vi "UMLEditor BusyDialog.vi"(1 "ToDialog":refnum<user-event>, 2 "FromDialog":refnum<queue>, 5 "error in":errorcluster) -> (19 "error out":errorcluster)   [LabVIEW 2012]
panel:
  out "StatusOut":string
  in  "Abort":bool
  out "TitleOut":string
  out "LoadedVIs":i32(graph)
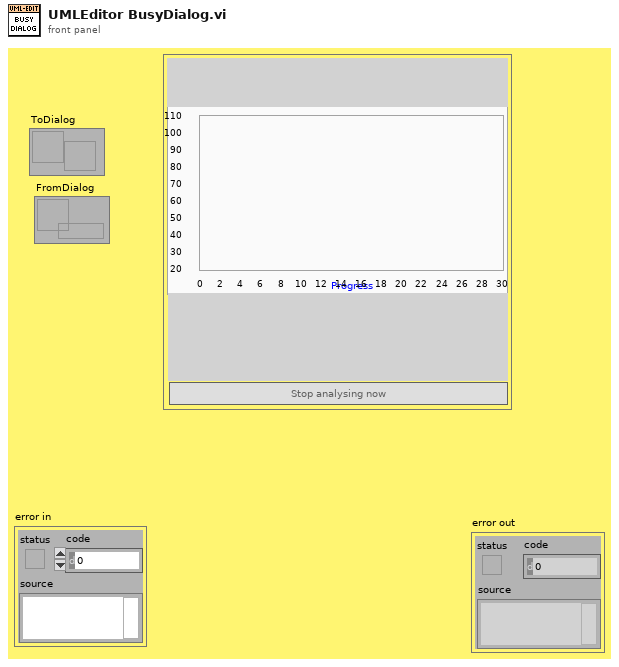
[diagram p1: front panel]
types:
  T1 = cluster{"CommandArgument":string, "Active":bool, "VIsInMem":i32, "ShowVIs":bool, "Event":refnum<event-registration>}
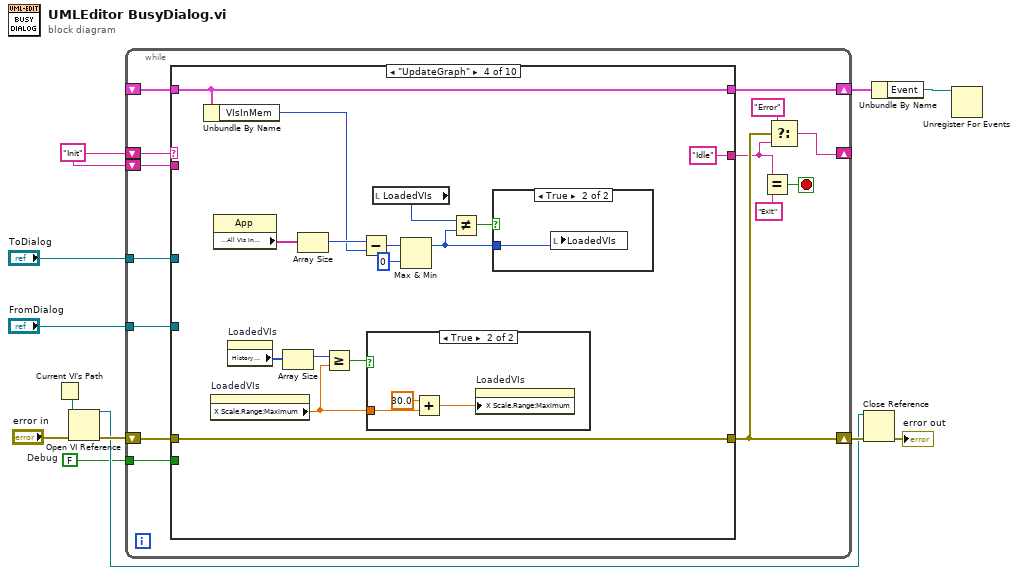
[diagram p0: block diagram]
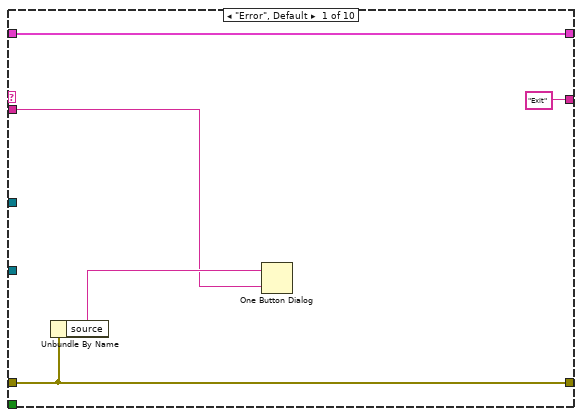
[diagram p2: hidden frame]
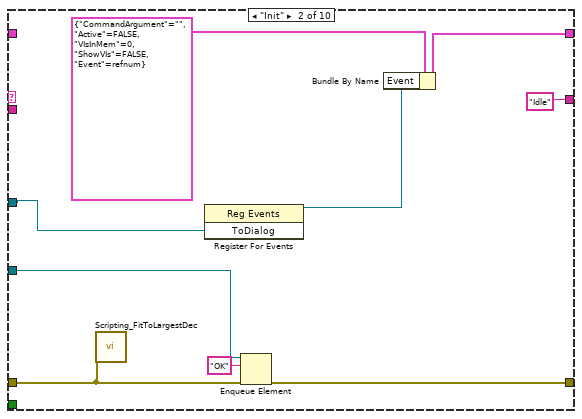
[diagram p3: hidden frame]
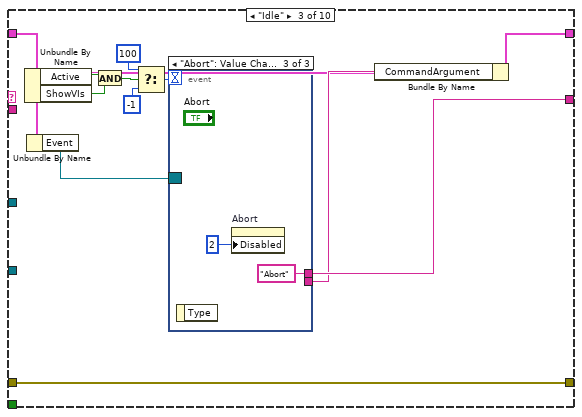
[diagram p4: hidden frame]
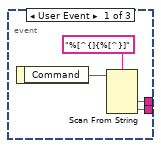
[diagram p5: hidden frame]
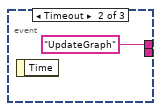
[diagram p6: hidden frame]
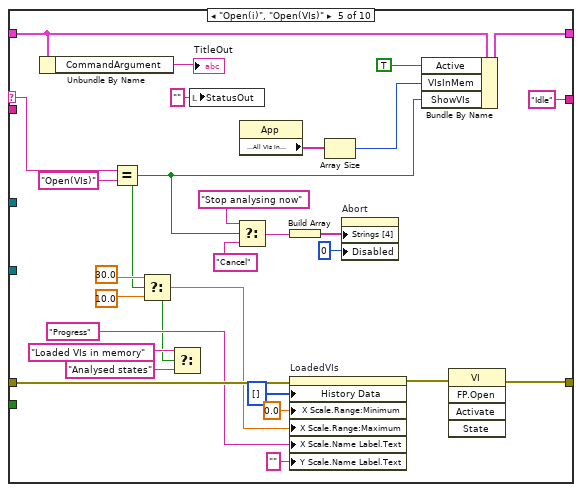
[diagram p9: hidden frame]
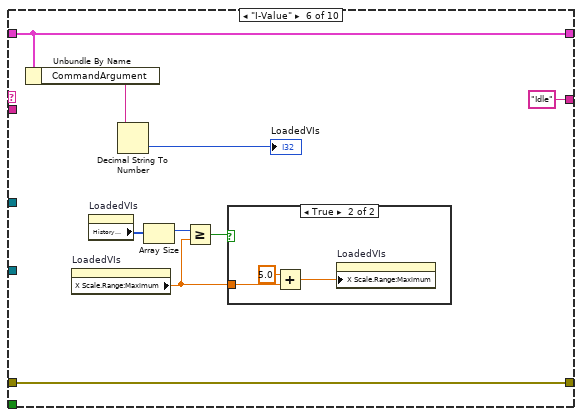
[diagram p10: hidden frame]
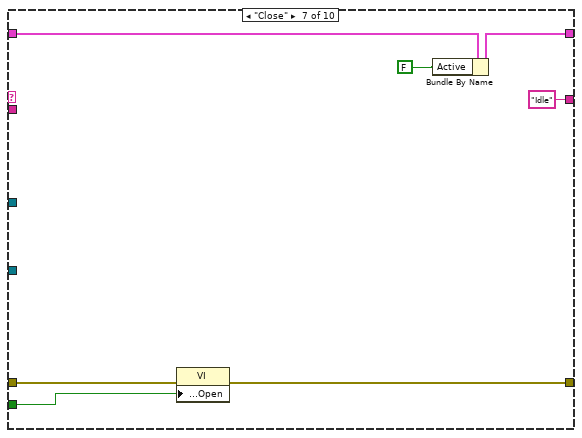
[diagram p12: hidden frame]
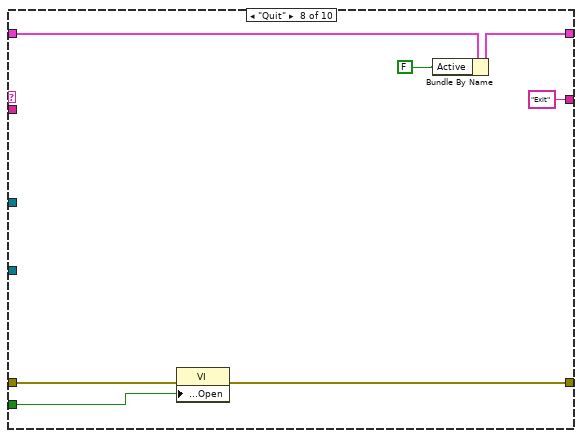
[diagram p13: hidden frame]
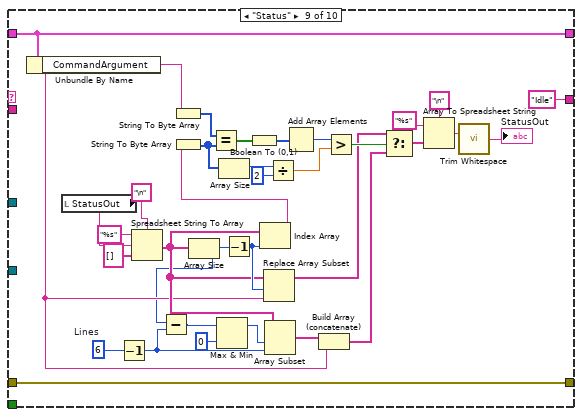
[diagram p14: hidden frame]
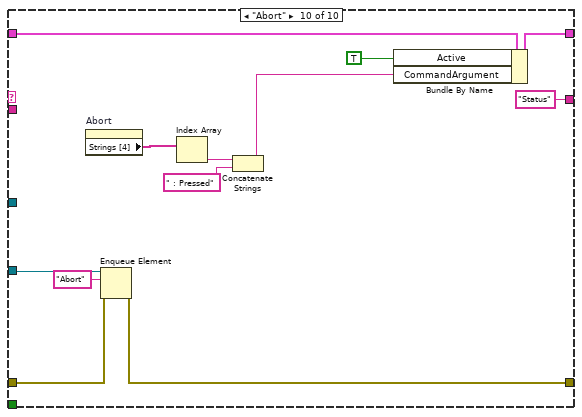
[diagram p15: hidden frame]
diagram:
  w3 = FALSE  # Debug
  w4 = "Init"
  n1 = Current VI's Path() -> (path=w5:path)
  n2 = Open VI Reference(vi path=w5, error in (no error)="error in") -> (vi reference=w8:refnum<vi>, error out=w11:errorcluster)  [unwired: 4 out]
  n3 = while {
    shift-right: [w23] -> _
    shift-left: w4 -> [w26]
    shift-right: [w24] -> w10
    shift-left: w11 -> [w25]
    tunnel: "FromDialog" -> [w18]
    tunnel: "ToDialog" -> [w17]
    shift-right: [w15] -> w2
    shift-left: _ -> [w16]
    shift-left: w4 -> [w14]
    tunnel: w3 -> [w13]
    stop <- w19 stop-if-true
    n4 = case shown="\"UpdateGraph\"" w26 {
      selector: w26 -> [_ _ _ _ w95 _ _ _ _ _]
      tunnel: w25 -> [w28 w32 w43 w74 w99 w114 w125 w132 w165 w173]
      tunnel: [w28 w39 w43 w74 w80 w114 w124 w131 w165 w171] -> w24
      tunnel: ["Exit" "Idle" w52 "Idle" "Idle" "Idle" "Idle" "Exit" "Idle" "Status"] -> w21
      tunnel: w18 -> [_ w38 _ _ _ _ _ _ _ w174]
      tunnel: w17 -> [_ w36 _ _ _ _ _ _ _ _]
      tunnel: w16 -> [w30 _ w42 w64 w105 w112 w123 w130 w164 w178]
      tunnel: [w30 w34 w51 w64 w103 w112 w121 w128 w164 w176] -> w15
      tunnel: w14 -> [w27 _ _ _ _ _ _ _ _ _]
      tunnel: w13 -> [_ _ _ _ _ _ w119 w126 _ _]
      frame "Error", Default {
        n5 = Unbundle By Name(w28) -> ("source"=w29:string)
        n6 = One Button Dialog(message=w29, button name ("OK")=w27) -> ()  [unwired: 1 out]
      }
      frame "Init" {
        n7 = call <resource>:"Scripting_FitToLargestDec.vi"("error in (no error)"=w32) -> ()  [unwired: 5 in, 2 out]
        n8 = register-events(w36) -> (reference out=w33:refnum<event-registration>)  [unwired: 2 in, 1 out]
        n9 = Enqueue Element(queue=w38, element="OK", error in (no error)=w32) -> (error out=w39:errorcluster)  [unwired: 3 out]
        n10 = Bundle By Name(cluster=T1 {"CommandArgument"="", "Active"=FALSE, "VIsInMem"=0, "ShowVIs"=FALSE, "Event"=refnum}, "Event"=w33) -> (w34:T1)
      }
      frame "Idle" {
        n11 = Unbundle By Name(w42) -> ("Active"=w45:bool, "ShowVIs"=w44:bool)
        n12 = Unbundle By Name(w42) -> ("Event"=w41:refnum<event-registration>)
        n13 = And(x=w45, y=w44) -> (x .and. y?=w46:bool)
        n14 = Select(t=100, s=w46, f=-1) -> (s? t:f=w49:i32)
        n15 = event shown="[2] \"Abort\": Value Change" {
          selector: w41 -> [_ _ _]
          dyn-events: _ -> [_ _ _]
          timeout: w49 -> [_ _ _]
          tunnel: [w55 "UpdateGraph" "Abort"] -> w52
          tunnel: [w54 _ _] -> w50
          event User Event {
            n16 = event-data() -> ("Command"=w53:string)  [unwired: 1 out]
            n17 = Scan From String(format string="%[^{]{%[^}]", input string=w53) -> (output 1=w55:string, output 2=w54:string)  [unwired: 2 in, 5 out]
          }
          event Timeout {
            n18 = event-data() -> ()  [unwired: 2 out]
          }
          event "Abort": Value Change {
            n19 = event-data() -> ()  [unwired: 2 out]
            n20 = property on="Abort" class="Bool"("Disabled"=u8 2) -> ()  [unwired: 2 in, 2 out]
          }
        }
        n21 = Bundle By Name(cluster=w42, "CommandArgument"=w50) -> (w51:T1)
      }
      frame "UpdateGraph" {
        n22 = Unbundle By Name(w64) -> ("VIsInMem"=w71:i32)
        n23 = property on="LoadedVIs" class="WFChart (strict)"() -> ("X Scale.Range:Maximum"=w60:dbl)  [unwired: 2 in, 2 out]
        n24 = property class="App"() -> ("Application:All VIs In Memory"=w73:string[])  [unwired: 2 in, 2 out]
        n25 = property on="LoadedVIs" class="WFChart (strict)"() -> ("History Data"=w63:i32[])  [unwired: 2 in, 2 out]
        n26 = Array Size(array=w63) -> (size(s)=w62:i32)
        n27 = Array Size(array=w73) -> (size(s)=w72:i32)
        n28 = Greater Or Equal?(x=w62, y=w60) -> (x >= y?=w61:bool)
        n29 = Subtract(x=w72, y=w71) -> (x-y=w70:i32)
        n30 = case shown="True" w61 {
          tunnel: w60 -> [_ w77]
          frame False {
          }
          frame True {
            n31 = Add(x=30.0, y=w77) -> (x+y=w75:dbl)
            n32 = property on="LoadedVIs" class="WFChart (strict)"("X Scale.Range:Maximum"=w75) -> ()  [unwired: 2 in, 2 out]
          }
        }
        n33 = local read "LoadedVIs"() -> (w68:i32)
        n34 = Max & Min(x=w70, y=0) -> (max(x,y)=w66:i32)  [unwired: 1 out]
        n35 = Not Equal?(x=w68, y=w66) -> (x != y?=w67:bool)
        n36 = case shown="True" w67 {
          tunnel: w66 -> [_ w78]
          frame False {
          }
          frame True {
            n37 = local write "LoadedVIs"(w78) -> ()
          }
        }
      }
      frame "Open(i)", "Open(VIs)" {
        n38 = Unbundle By Name(w105) -> ("CommandArgument"=→"TitleOut":string)
        n39 = Equal?(x=w95, y="Open(VIs)") -> (x = y?=w85:bool)
        n40 = Select(t=30.0 ("X Scale.Range:Maximum"), s=w85, f=10.0 ("X Scale.Range:Maximum")) -> (s? t:f=w91:dbl)
        n41 = Select(t="Loaded VIs in memory" ("StatusOut"), s=w85, f="Analysed states" ("StatusOut")) -> ()  [unwired: 1 out]
        n42 = local write "StatusOut"("" ("StatusOut")) -> ()
        n43 = Select(t="Stop analysing now" ("StatusOut"), s=w85, f="Cancel" ("StatusOut")) -> (s? t:f=w86:string)
        n44 = property class="App"() -> ("Application:All VIs In Memory"=w101:string[])  [unwired: 2 in, 2 out]
        n45 = Build Array(w86) -> (w87:string[])
        n46 = property on="LoadedVIs" class="WFChart (strict)"(error in=w99, "History Data"=i32[] [], "X Scale.Range:Minimum"=0.0, "X Scale.Range:Maximum"=w91, "X Scale.Name Label.Text"="Progress" ("StatusOut"), "Y Scale.Name Label.Text"="") -> (error out=w81:errorcluster)  [unwired: 1 in, 1 out]
        n47 = Array Size(array=w101) -> (size(s)=w100:i32)
        n48 = property on="Abort" class="Bool"("Strings [4]"=w87, "Disabled"=u8 0) -> ()  [unwired: 2 in, 2 out]
        n49 = Bundle By Name(cluster=w105, "Active"=TRUE, "VIsInMem"=w100, "ShowVIs"=w85) -> (w103:T1)
        n50 = invoke class="VI" method="FP.Open"(error in=w81) -> (error out=w80:errorcluster)  [unwired: 4 in, 4 out]
      }
      frame "I-Value" {
        n51 = Unbundle By Name(w112) -> ("CommandArgument"=w115:string)
        n52 = property on="LoadedVIs" class="WFChart (strict)"() -> ("X Scale.Range:Maximum"=w108:dbl)  [unwired: 2 in, 2 out]
        n53 = property on="LoadedVIs" class="WFChart (strict)"() -> ("History Data"=w111:i32[])  [unwired: 2 in, 2 out]
        n54 = Decimal String To Number(string=w115) -> (number=→"LoadedVIs":i32)  [unwired: 3 out]
        n55 = Array Size(array=w111) -> (size(s)=w110:i32)
        n56 = Greater Or Equal?(x=w110, y=w108) -> (x >= y?=w109:bool)
        n57 = case shown="True" w109 {
          tunnel: w108 -> [_ w118]
          frame False {
          }
          frame True {
            n58 = Add(x=5.0, y=w118) -> (x+y=w116:dbl)
            n59 = property on="LoadedVIs" class="WFChart (strict)"("X Scale.Range:Maximum"=w116) -> ()  [unwired: 2 in, 2 out]
          }
        }
      }
      frame "Close" {
        n60 = property class="VI"(error in=w125, "Front Panel Window:Open"=w119) -> (error out=w124:errorcluster)  [unwired: 1 in, 1 out]
        n61 = Bundle By Name(cluster=w123, "Active"=FALSE) -> (w121:T1)
      }
      frame "Quit" {
        n62 = property class="VI"(error in=w132, "Front Panel Window:Open"=w126) -> (error out=w131:errorcluster)  [unwired: 1 in, 1 out]
        n63 = Bundle By Name(cluster=w130, "Active"=FALSE) -> (w128:T1)
      }
      frame "Status" {
        w135 = 6  # Lines
        n64 = Unbundle By Name(w164) -> ("CommandArgument"=w139:string)
        n65 = local read "StatusOut"() -> (w160:string)
        n66 = Decrement(x=w135) -> (x-1=w134:i32)
        n67 = Spreadsheet String To Array(delimiter (Tab)="\n", format string="%s", spreadsheet string=w160, array type (2D Dbl)=string[] []) -> (array=w147:string[])
        n68 = String To Byte Array(string=w139) -> (unsigned byte array=w156:u8[])
        n69 = Array Size(array=w147) -> (size(s)=w136:i32)
        n70 = Subtract(x=w136, y=w134) -> (x-y=w133:i32)
        n71 = Max & Min(x=w133, y=0) -> (max(x,y)=w138:i32)  [unwired: 1 out]
        n72 = Decrement(x=w136) -> (x-1=w149:i32)
        n73 = Index Array(array=w147, index=w149) -> (element=w157:string)
        n74 = String To Byte Array(string=w157) -> (unsigned byte array=w155:u8[])
        n75 = Equal?(x=w156, y=w155) -> (x = y?=w159:bool[])
        n76 = Array Size(array=w155) -> (size(s)=w153:i32)
        n77 = Boolean To (0,1)(Boolean=w159) -> (0, 1=w158:i16[])
        n78 = Replace Array Subset(array=w147, new element=w139, index=w149) -> (w148:string[])
        n79 = Array Subset(array=w147, index=w138, length=w134) -> (w141:string[])
        n80 = Divide(x=w153, y=2) -> (x/y=w151:dbl)
        n81 = Add Array Elements(numeric array=w158) -> (sum=w154:i16)
        n82 = Build Array (concatenate)(w141, w139) -> (w140:string[])
        n83 = Greater?(x=w154, y=w151) -> (0:w150:bool)
        n84 = Select(t=w148, s=w150, f=w140) -> (s? t:f=w146:string[])
        n85 = Array To Spreadsheet String(delimiter (Tab)="\n", array=w146, 3:"%s" ("format string")) -> (spreadsheet string=w143:string)
        n86 = call <vilib>:"Trim Whitespace.vi"("string"=w143) -> ("trimmed string"=→"StatusOut":string)  [unwired: 1 in]
      }
      frame "Abort" {
        n87 = property on="Abort" class="Bool"() -> ("Strings [4]"=w170:string[])  [unwired: 2 in, 2 out]
        n88 = Enqueue Element(queue=w174, element="Abort", error in (no error)=w173) -> (error out=w171:errorcluster)  [unwired: 3 out]
        n89 = Index Array(array=w170) -> (element=w169:string)  [unwired: 1 in]
        n90 = Concatenate Strings(w169, " : Pressed" ("string")) -> (w167:string)
        n91 = Bundle By Name(cluster=w178, "Active"=TRUE, "CommandArgument"=w167) -> (w176:T1)
      }
    }
    n92 = Equal?(x=w21, y="Exit") -> (x = y?=w19:bool)
    n93 = Select(t="Error", s=w24, f=w21) -> (s? t:f=w23:string)
  }
  n94 = Close Reference(reference=w8, error in (no error)=w10) -> (error out=→"error out":errorcluster)
  n95 = Unbundle By Name(w2) -> ("Event"=w1:refnum<event-registration>)
  n96 = Unregister For Events(event registration refnum=w1) -> ()  [unwired: 1 in, 1 out]
